vi "NF LI56xx dvr qDATA COUNT.vi"(8 "error in":errorcluster caption="error in (no error)" {"code" format="%.0x"}, 10 "set data buffer":enum16{"BUF1", "BUF2", "BUF3"}(ring), 11 "VISA resource name":refnum<visa-resource-name>) -> (0 "error out":errorcluster {"code" format="%.0x"}, 2 "query sampling points":string, 3 "VISA resource name copy":refnum<visa-resource-name>)   [LabVIEW 2019]
doc: "Queries the number of data sampling points recorded in the measurement data buffer."
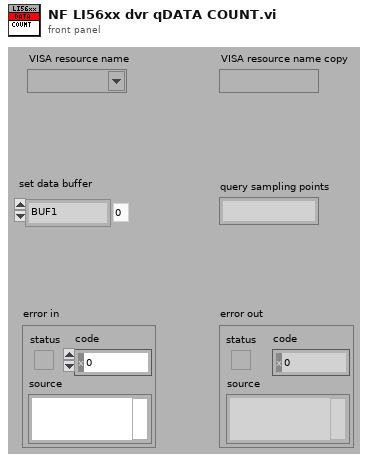
[diagram p1: front panel]
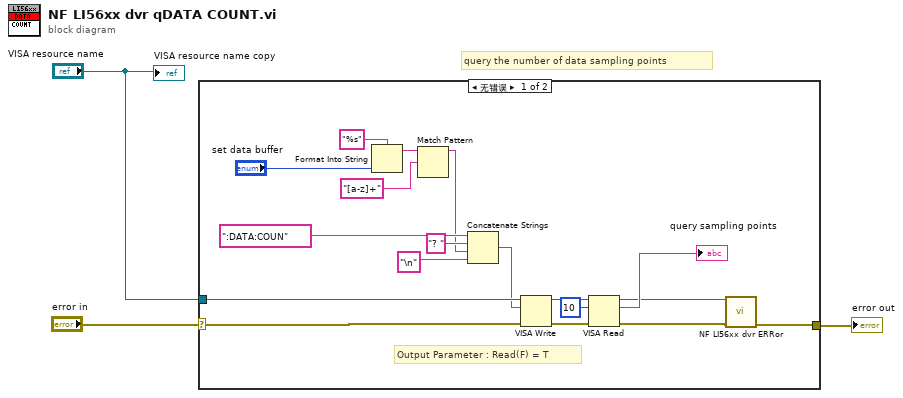
[diagram p0: block diagram]
diagram:
  # "query the number of data sampling points"
  n1 = case shown="无错误" "error in" {
    selector: "error in" -> [w21 w22]
    tunnel: [w15 w22] -> w3
    tunnel: "VISA resource name" -> [w20 _]
    frame No Error {
      # "Output Parameter : Read(F) = T"
      n2 = Format Into String(format string="%s", "set data buffer") -> (resulting string=w7:string)  [unwired: 2 in, 1 out]
      n3 = Match Pattern(string=w7, regular expression="[a-z]+") -> (before substring=w5:string)  [unwired: 1 in, 3 out]
      n4 = Concatenate Strings(":DATA:COUN" ("•¶Žš—ñ"), "? " ("Œ`Ž®•¶Žš—ñ"), w5, "\n" ("Œ`Ž®•¶Žš—ñ")) -> (w9:string)
      n5 = VISA Write(VISA resource name=w20, write buffer=w9, error in (no error)=w21) -> (VISA resource name out=w12:refnum<visa-resource-name>, error out=w13:errorcluster)  [unwired: 1 out]
      n6 = VISA Read(VISA resource name=w12, byte count=u32 10 ("バイトカウント（0）"), error in (no error)=w13) -> (VISA resource name out=w17:refnum<visa-resource-name>, read buffer=→"query sampling points":string, error out=w16:errorcluster)  [unwired: 1 out]
      n7 = call "NF LI56xx dvr ERRor.vi"("VISA resource name"=w17, "error in (no error)"=w16) -> ("error out"=w15:errorcluster)  [unwired: 10 in, 3 out]
    }
    frame Error {
    }
  }
  "error out" <- w3
  "VISA resource name copy" <- "VISA resource name"
